vi "read_id.vi"(8 "error in (no error)":errorcluster, 11 "VISA resource name in":refnum<visa-resource-name>) -> (0 "error out":errorcluster, 2 "ID string":string, 3 "VISA resource name out":refnum<visa-resource-name>)   [LabVIEW 2009]
uses:
  <vilib>/Instr/_visa.llb/VISA Configure Serial Port (Instr).vi
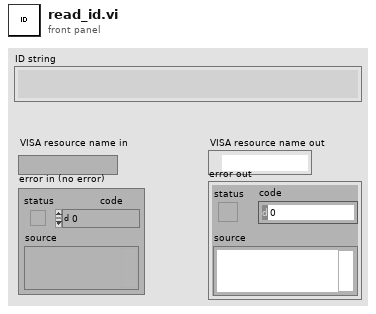
[diagram p1: front panel]
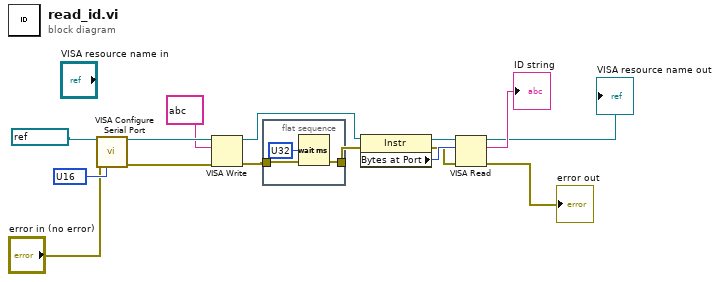
[diagram p0: block diagram]
diagram:
  w14 = u16 ? items=["1.0", "1.5", "2.0"] ("stop bits (10: 1 bit)")
  n1 = call-poly "VISA Configure Serial Port"("VISA resource name"=refnum<visa-resource-name> ?, "error in (no error)"="error in (no error)", "stop bits (10: 1 bit)"=w14) -> ("VISA resource name out"=w13:refnum<visa-resource-name>, "error out"=w12:errorcluster)  [unwired: 11 in]
  n2 = VISA Write(VISA resource name=w13, write buffer=string ?, error in (no error)=w12) -> (VISA resource name out=w3:refnum<visa-resource-name>, error out=w5:errorcluster)  [unwired: 1 out]
  n3 = flat-sequence {
    tunnel: w5 -> [w17]
    tunnel: [w17] -> w4
    frame #0 {
      n4 = Wait (ms)(milliseconds to wait=u32 ?) -> ()  [unwired: 1 out]
    }
  }
  n5 = property class="Instr"(reference=w3, error in=w4) -> (reference out=w7:refnum<visa-resource-name>, error out=w6:errorcluster, "Bytes at Port"=w8:u32)
  n6 = VISA Read(VISA resource name=w7, byte count=w8, error in (no error)=w6) -> (VISA resource name out=→"VISA resource name out":refnum<visa-resource-name>, read buffer=→"ID string":string, error out=→"error out":errorcluster)  [unwired: 1 out]
